vi "Write VI-Ref.vi"(8 "error in (no error)":errorcluster, 10 "VI-Ref":refnum<vi>, 11 "Quick-GUI-Update in":refnum<class "Quick-GUI-Update.lvclass">) -> (0 "error out":errorcluster, 3 "Quick-GUI-Update out":refnum<class "Quick-GUI-Update.lvclass">)   [LabVIEW 2020, in "Easy GUI Operation.lvlib" / "Quick-GUI-Update.lvclass"]
uses:
  Quick-GUI-Update.lvclass
  Quick-GUI-Update.lvclass/Quick-GUI-Update.ctl
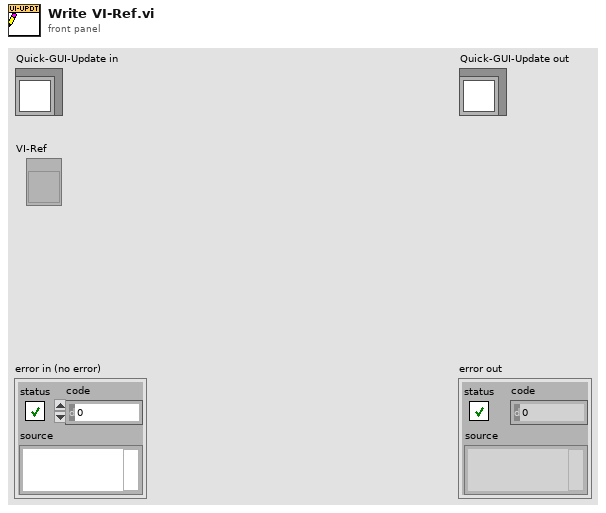
[diagram p1: front panel]
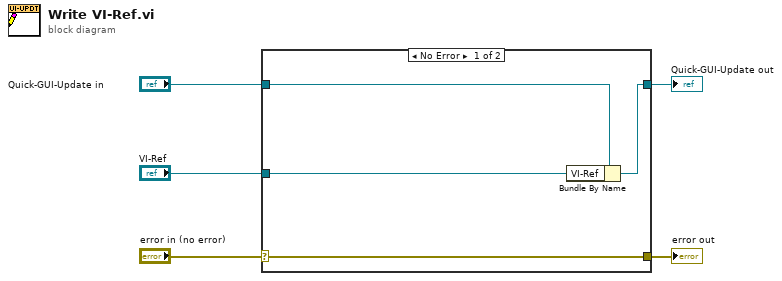
[diagram p0: block diagram]
diagram:
  n1 = case shown="No Error" "error in (no error)" {
    selector: "error in (no error)" -> [w9 w10]
    tunnel: [w9 w10] -> w4
    tunnel: [w7 w11] -> w2
    tunnel: "Quick-GUI-Update in" -> [w8 w11]
    tunnel: "VI-Ref" -> [w6 _]
    frame No Error {
      n2 = Bundle By Name(cluster=w8, "VI-Ref"=w6) -> (w7:refnum<class "Quick-GUI-Update.lvclass">)
    }
    frame Error {
    }
  }
  "error out" <- w4
  "Quick-GUI-Update out" <- w2
